vi "Write add enable channel.vi"(8 "error in (no error)":errorcluster, 10 "add enable channel":bool, 11 "TDMS datalogger configuration in":refnum<class "TDMS datalogger configuration.lvclass">) -> (0 "error out":errorcluster, 3 "TDMS datalogger configuration out":refnum<class "TDMS datalogger configuration.lvclass">)   [LabVIEW 2015, in "TDMS datalogger configuration.lvclass"]
uses:
  TDMS datalogger configuration.lvclass
  TDMS datalogger configuration.lvclass/TDMS datalogger configuration.ctl
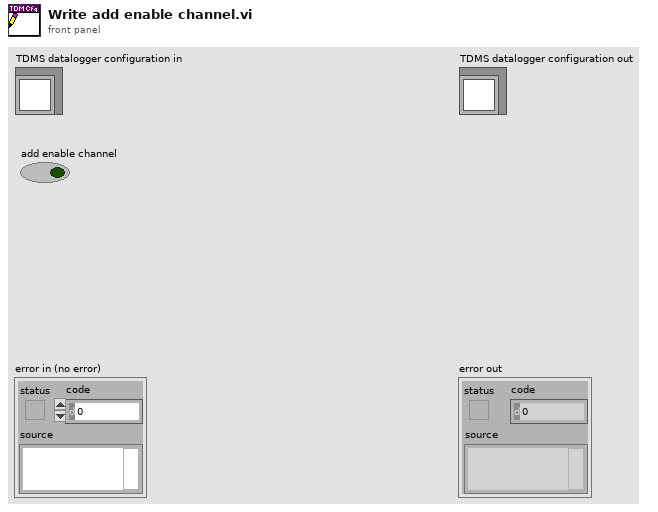
[diagram p1: front panel]
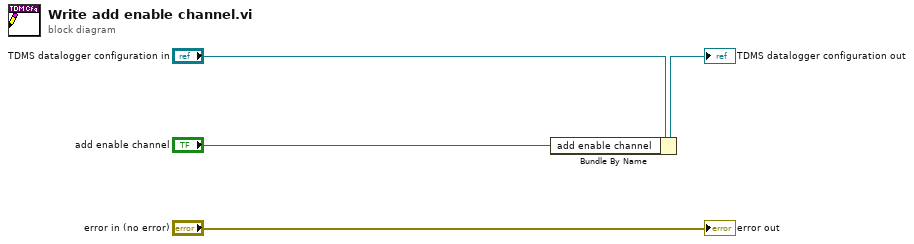
[diagram p0: block diagram]
diagram:
  n1 = Bundle By Name(cluster="TDMS datalogger configuration in", "add enable channel"="add enable channel") -> (→"TDMS datalogger configuration out":refnum<class "TDMS datalogger configuration.lvclass">)
  "error out" <- "error in (no error)"
